vi "Configure Overlay Cluster_Galvo_Reso.vi"(8 "Error In":errorcluster, 10 "Overlay Control Reference":refnum<vi>, 11 "Overlay Control Type":string) -> (0 "Error Out":errorcluster)   [LabVIEW 2012]
doc: "SciScan 1.2 160622"
uses:
  Custom Control and Typedefs/Overlay Control.ctl
  <vilib>/Utility/miscctls.llb/LVFormatAndPrecisionTypeDef.ctl
panel:
  # "Red (Current Image)"
  # "Green (Saved Image)"
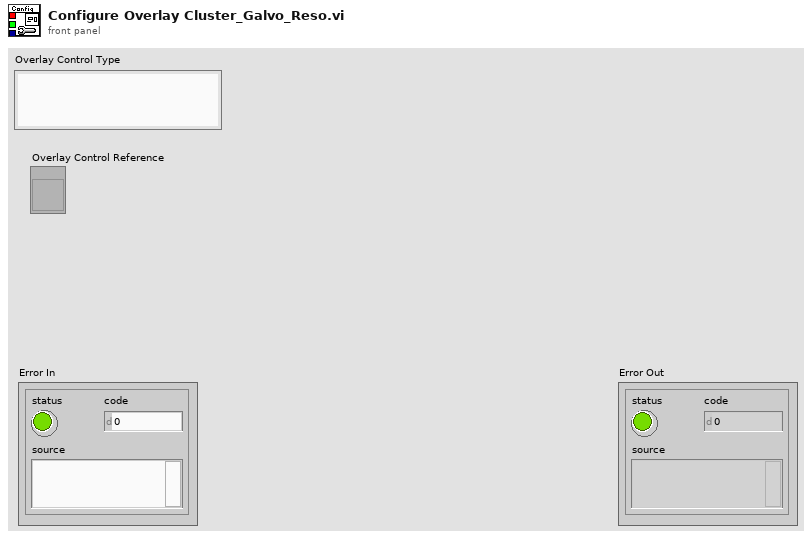
[diagram p1: front panel]
types:
  T1 = typedef "LVFormatAndPrecisionTypeDef.ctl" = cluster{"Format":u8, "Precision":u8}
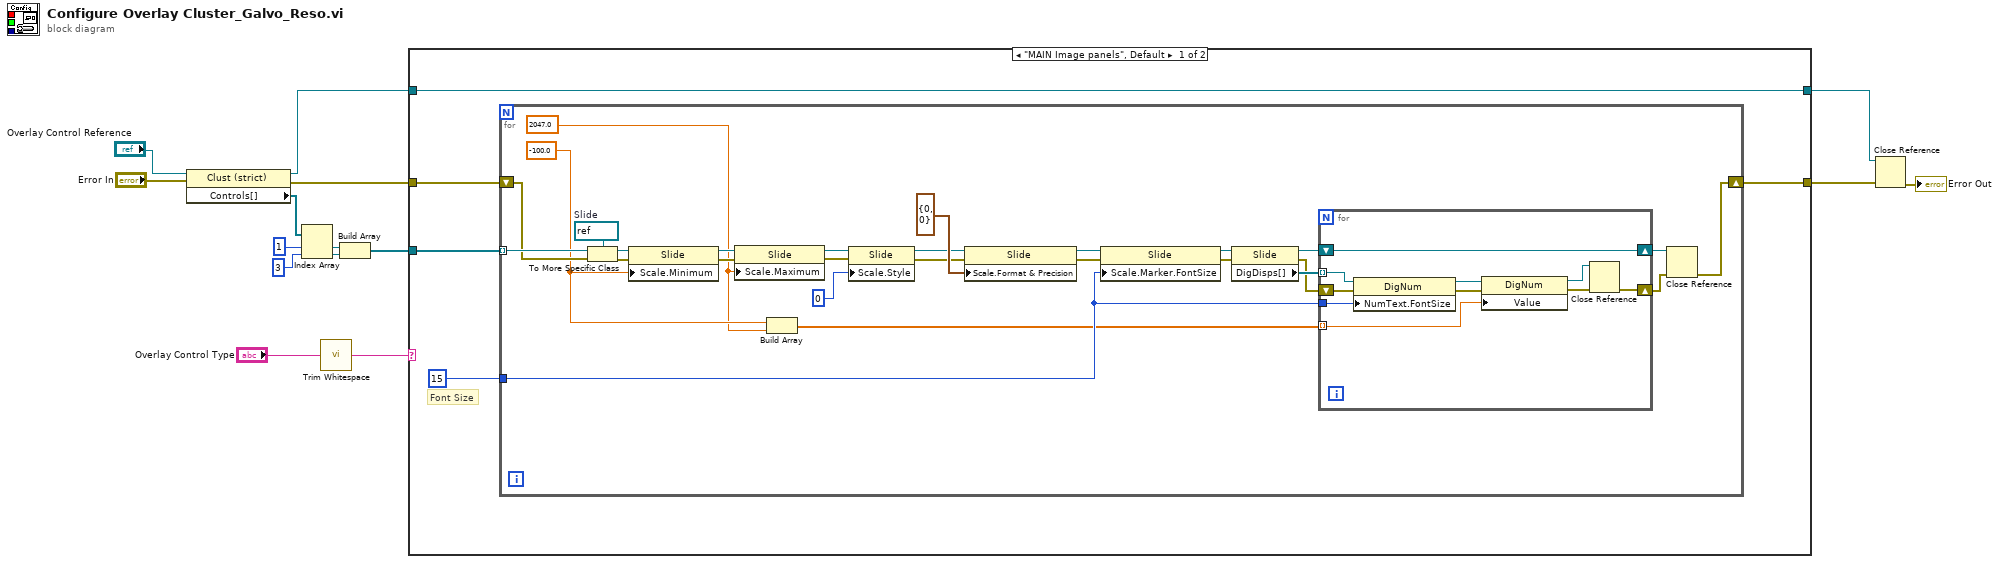
[diagram p0: block diagram]
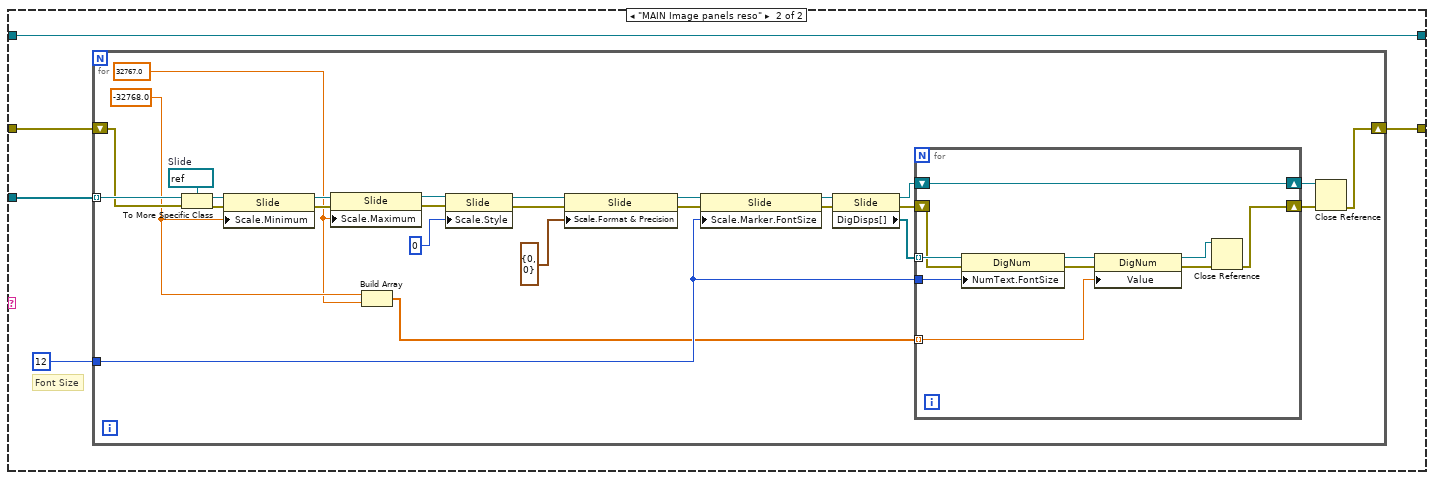
[diagram p2: hidden frame]
diagram:
  n1 = property class="Clust (strict)"(reference="Overlay Control Reference", error in="Error In") -> (reference out=w4:refnum<vi>, error out=w7:errorcluster, "Controls[]"=w9:refnum<vi>[])
  n2 = Index Array(array=w9, index #1=1 ("index"), index #2=3 ("index")) -> (element #1=w12:refnum<vi>, element #2=w13:refnum<vi>)
  n3 = call <vilib>:"Trim Whitespace.vi"("string"="Overlay Control Type") -> ("trimmed string"=w14:string)  [unwired: 1 in]
  n4 = Build Array(w12, w13) -> (w8:refnum<vi>[])
  n5 = case shown="\"MAIN Image panels\", Default" w14 {
    tunnel: [w19 w61] -> w2
    tunnel: w8 -> [w18 w60]
    tunnel: w7 -> [w17 w59]
    tunnel: w4 -> [w16 w58]
    tunnel: [w16 w58] -> w3
    frame "MAIN Image panels", Default {
      # "Font Size"
      n6 = for {
        tunnel: u32 15 ("Scale.Marker.Font:Size") -> [w38]
        tunnel: w18 -> [w35] mode=indexing
        shift-right: [w26] -> w19
        shift-left: w17 -> [w34]
        w46 = refnum<vi> refnum  # Slide
        w32 = 2047.0
        w33 = -100.0
        n7 = To More Specific Class(target class=w46, reference=w35, error in=w34) -> (specific class reference=w47:refnum<vi>, error out=w45:errorcluster)
        n8 = property class="Slide"(reference=w47, error in=w45, "Scale.Minimum"=w33) -> (reference out=w44:refnum<vi>, error out=w43:errorcluster)
        n9 = property class="Slide"(reference=w44, error in=w43, "Scale.Maximum"=w32) -> (reference out=w42:refnum<vi>, error out=w41:errorcluster)
        n10 = Build Array(w33, w32) -> (w31:dbl[])
        n11 = property class="Slide"(reference=w42, error in=w41, "Scale.Style"=u8 0 ("Scale.Display Format:Format")) -> (reference out=w24:refnum<vi>, error out=w23:errorcluster)
        n12 = property class="Slide"(reference=w24, error in=w23, "Scale.Format & Precision"=T1 {"Format"=0, "Precision"=0} ("Scale.Display Format")) -> (reference out=w22:refnum<vi>, error out=w21:errorcluster)
        n13 = property class="Slide"(reference=w22, error in=w21, "Scale.Marker.FontSize"=w38) -> (reference out=w37:refnum<vi>, error out=w36:errorcluster)
        n14 = property class="Slide"(reference=w37, error in=w36) -> (reference out=w29:refnum<vi>, error out=w30:errorcluster, "DigDisps[]"=w39:refnum<vi>[])
        n15 = for {
          tunnel: w39 -> [w57] mode=indexing
          tunnel: w38 -> [w56]
          tunnel: w31 -> [w50] mode=indexing
          shift-right: [w49] -> w27
          shift-left: w30 -> [w55]
          shift-right: [w48] -> w28
          shift-left: w29 -> [w48]
          n16 = property class="DigNum"(reference=w57, error in=w55, "NumText.FontSize"=w56) -> (reference out=w53:refnum<vi>, error out=w54:errorcluster)
          n17 = property class="DigNum"(reference=w53, error in=w54, "Value"=w50) -> (reference out=w51:refnum<vi>, error out=w52:errorcluster)
          n18 = Close Reference(reference=w51, error in (no error)=w52) -> (error out=w49:errorcluster)
        }
        n19 = Close Reference(reference=w28, error in (no error)=w27) -> (error out=w26:errorcluster)
      }
    }
    frame "MAIN Image panels reso" {
      # "Font Size"
      n20 = for {
        tunnel: u32 12 ("Scale.Marker.Font:Size") -> [w80]
        tunnel: w60 -> [w77] mode=indexing
        shift-right: [w68] -> w61
        shift-left: w59 -> [w76]
        w88 = refnum<vi> refnum  # Slide
        w74 = 32767.0
        w75 = -32768.0
        n21 = To More Specific Class(target class=w88, reference=w77, error in=w76) -> (specific class reference=w89:refnum<vi>, error out=w87:errorcluster)
        n22 = property class="Slide"(reference=w89, error in=w87, "Scale.Minimum"=w75) -> (reference out=w86:refnum<vi>, error out=w85:errorcluster)
        n23 = property class="Slide"(reference=w86, error in=w85, "Scale.Maximum"=w74) -> (reference out=w84:refnum<vi>, error out=w83:errorcluster)
        n24 = Build Array(w75, w74) -> (w73:dbl[])
        n25 = property class="Slide"(reference=w84, error in=w83, "Scale.Style"=u8 0 ("Scale.Display Format:Format")) -> (reference out=w67:refnum<vi>, error out=w64:errorcluster)
        n26 = property class="Slide"(reference=w67, error in=w64, "Scale.Format & Precision"=T1 {"Format"=0, "Precision"=0} ("Scale.Display Format")) -> (reference out=w65:refnum<vi>, error out=w63:errorcluster)
        n27 = property class="Slide"(reference=w65, error in=w63, "Scale.Marker.FontSize"=w80) -> (reference out=w79:refnum<vi>, error out=w78:errorcluster)
        n28 = property class="Slide"(reference=w79, error in=w78) -> (reference out=w72:refnum<vi>, error out=w71:errorcluster, "DigDisps[]"=w81:refnum<vi>[])
        n29 = for {
          tunnel: w81 -> [w98] mode=indexing
          tunnel: w80 -> [w99]
          tunnel: w73 -> [w97] mode=indexing
          shift-right: [w92] -> w70
          shift-left: w71 -> [w94]
          shift-right: [w91] -> w69
          shift-left: w72 -> [w91]
          n30 = property class="DigNum"(reference=w98, error in=w94, "NumText.FontSize"=w99) -> (reference out=w90:refnum<vi>, error out=w93:errorcluster)
          n31 = property class="DigNum"(reference=w90, error in=w93, "Value"=w97) -> (reference out=w95:refnum<vi>, error out=w96:errorcluster)
          n32 = Close Reference(reference=w95, error in (no error)=w96) -> (error out=w92:errorcluster)
        }
        n33 = Close Reference(reference=w69, error in (no error)=w70) -> (error out=w68:errorcluster)
      }
    }
  }
  n34 = Close Reference(reference=w3, error in (no error)=w2) -> (error out=→"Error Out":errorcluster)
